vi "Close.vi"(8 "error in (no error)":errorcluster, 11 "NetA_RSZVL in":refnum<class "NetA_RSZVL.lvclass">) -> (0 "error out":errorcluster)   [LabVIEW 2014, in "NetA_RSZVL.lvclass"]
uses:
  NetA_RSZVL.lvclass
  NetA_RSZVL.lvclass/NetA_RSZVL.ctl
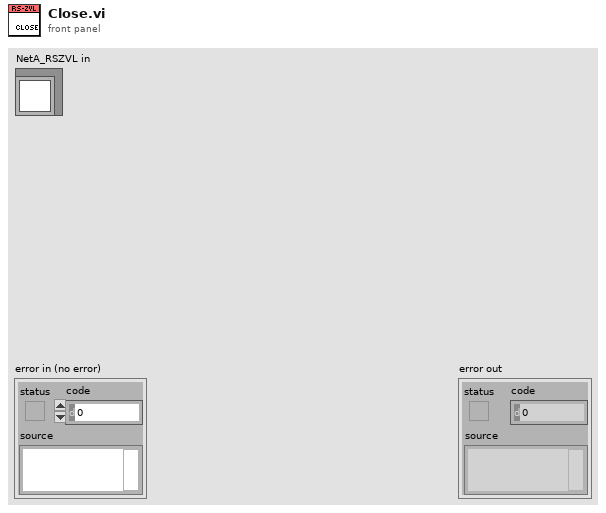
[diagram p1: front panel]
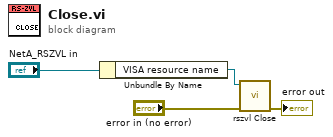
[diagram p0: block diagram]
diagram:
  n1 = Unbundle By Name("NetA_RSZVL in") -> ("VISA resource name"=w2:refnum<visa-resource-name>)
  n2 = call "rszvl Close.vi"("error in (no error)"="error in (no error)", "VISA resource name"=w2) -> ("error out"=→"error out":errorcluster)  [unwired: 9 in]
